vi "CRYProject Editor PART TS Write.vi"(7 "Channels":i32=2, 9 "Version":u16=1, 11 "pSaveName":path) -> (0 "Is Replace?":bool, 1 "SequenceFilepathOut":path, 2 "Sequence NameOut":string, 3 "status":bool, 4 "Flatten Doc Data":string, 5 "Flatten Curve Data":string)   [LabVIEW 2013]
uses:
  Control/CRYSequence Cluster.ctl
  CRYProject Editor Global.vi
  CRYSystem/Misc/SubVI/CRYMisc vis settings global.vi
  CRYMainGlobal.vi
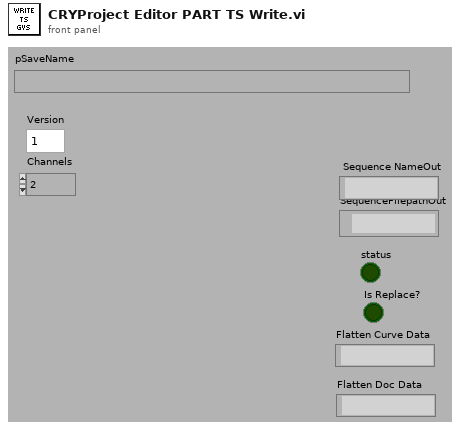
[diagram p1: front panel]
types:
  T1 = enum16{"New", "Open", "Close", "Close Data View Window Only", "Change", "Save", "Save for close"}
  T2 = typedef "CRYSequence Cluster.ctl" = cluster{"EditStepName":string, "Trimmed string array":string, "Flattened CurveData":string, "Document Data":string, "EditStepNo":u16, "Operator Start File":path, "Sequence Type":string, "Sequence Language":string, "Sequence Work State":string}
  T3 = enum16{"open", "replace", "create", "open or create", "replace or create", "replace or create with confirmation"}
  T4 = typedef "CRYTS.ctl" = cluster{"No.TS":u16, "TS File Path":path, "TS Name":string, "EditStepName":string, "Steps":T5[], "New State":bool, "Change State":bool, "Flattened CurveLib Data":string, "Document Data":string, "EditStepNo":u16, "Operator Start File":string, "Sequence Type":string, "Sequence Language":string}
  T5 = typedef "CRYStep.ctl" = cluster{"No.VI":i32, "Category":string, "StepName":string, "Seq setup flattened":string, "Comment":string, "Steps config.":bool[], "Jump config":i32[], "Start":dbl, "Increment":dbl, "Name":string, "Unit":string, "Y data":u16, "Y prefix":string, "Y dB ref":dbl, "Y unit":string, "Repeat State Array":cluster{"Start":dbl, "Increment":dbl, "Count":i32, "Num":i32}[]}
  T6 = enum32{"English", "Chinese", "Korean", "Japanese", "Russian", "Chinese traditional"}
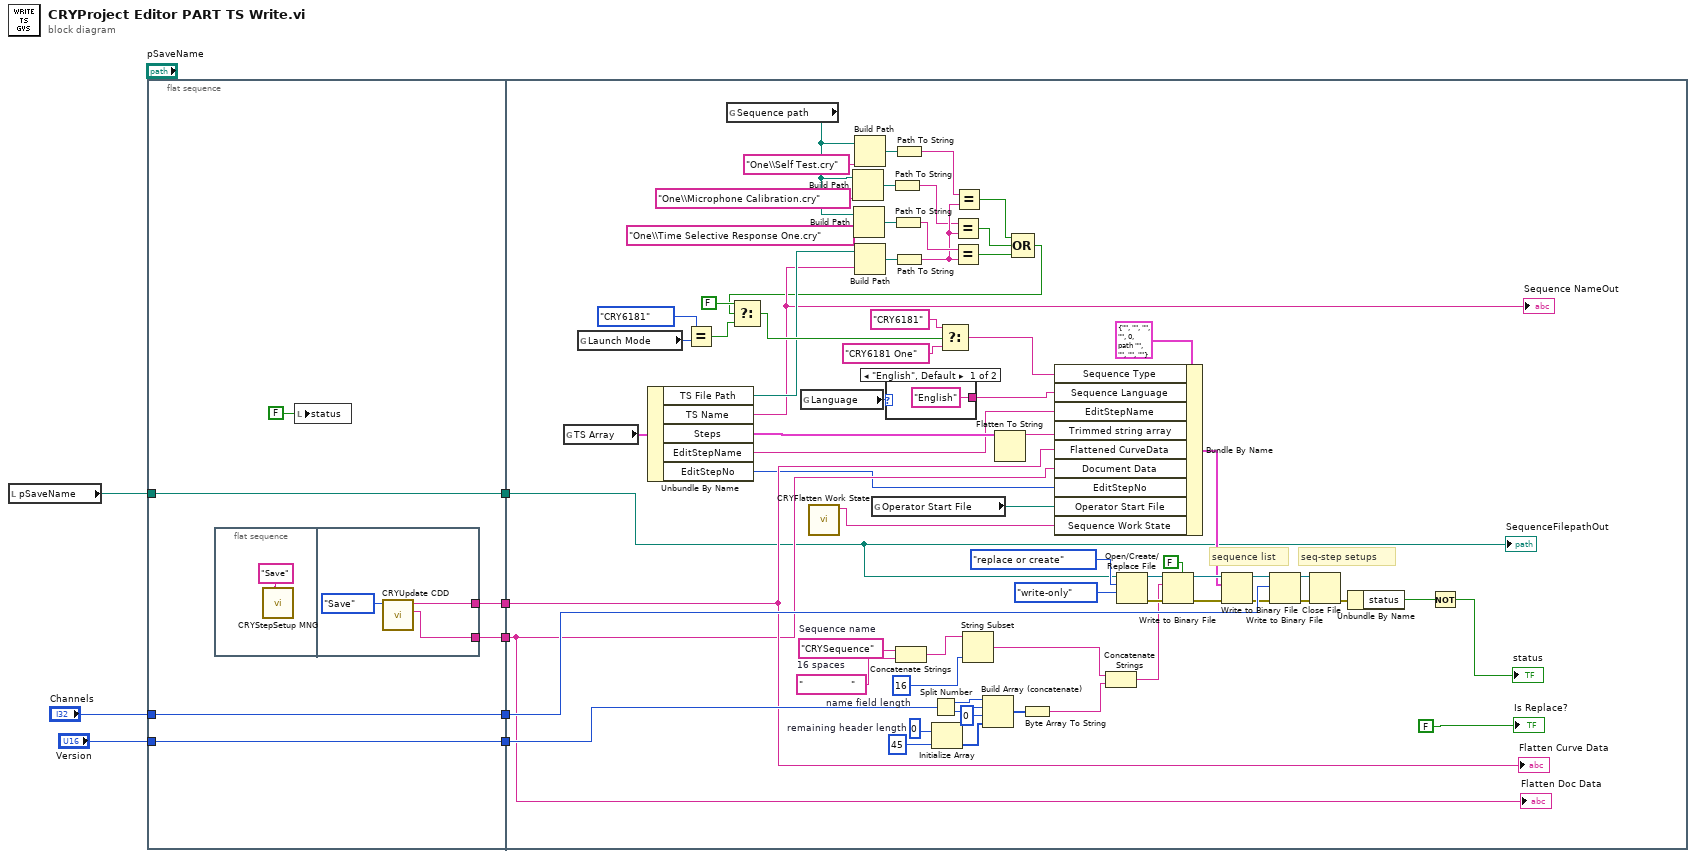
[diagram p0: block diagram]
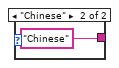
[diagram p2: hidden frame]
diagram:
  n1 = local read "pSaveName"() -> (w6:path)
  n2 = flat-sequence {
    tunnel: w6 -> [w12]
    tunnel: "Version" -> [w13]
    tunnel: "Channels" -> [w14]
    tunnel: [w14] -> w5
    tunnel: [w13] -> w4
    tunnel: [w10] -> w3
    tunnel: [w9] -> w2
    tunnel: [w12] -> w1
    tunnel: w5 -> [w88]
    tunnel: w4 -> [w87]
    tunnel: w3 -> [w84]
    tunnel: w2 -> [w83]
    tunnel: w1 -> [w51]
    frame #0 {
      n3 = flat-sequence {
        tunnel: [w16] -> w10
        tunnel: [w17] -> w9
        frame #0 {
          n4 = call "CRYStepSetup MNG.vi"("sAction"="Save" ("Option")) -> ()  [unwired: 9 in, 2 out]
        }
        frame #1 {
          n5 = call "CRYUpdate CDD.vi"("Signal"=T1."Save") -> ("Document Data Out"=w17:string, "Flatten Data Out"=w16:string)  [unwired: 2 in, 7 out]
        }
      }
      n6 = local write "status"(FALSE ("status")) -> ()
    }
    frame #1 {
      w63 = 16  # name field length
      w64 = "                "  # 16 spaces
      w65 = "CRYSequence"  # Sequence name
      w73 = 45  # remaining header length
      # "sequence list"
      # "seq-step setups"
      n7 = global read "CRYProject Editor Global.vi" "TS Array"() -> (w52:T4)
      n8 = global read "CRYMainGlobal.vi" "Launch Mode"() -> (w47:enum32{"CRY6181", "CRY6181 One"})
      n9 = Unbundle By Name(w52) -> ("TS File Path"=w37:path, "TS Name"=w36:string, "Steps"=w55:T5[], "EditStepName"=w53:string, "EditStepNo"=w50:u16)
      "Sequence NameOut" <- w36
      n10 = Equal?(x=enum32{"CRY6181", "CRY6181 One"}."CRY6181", y=w47) -> (x = y?=w44:bool)
      n11 = global read "CRYMainGlobal.vi" "Sequence path"() -> (w30:path)
      n12 = global read "CRYMainGlobal.vi" "Language"() -> (w22:T6)
      n13 = call "CRYFlatten Work State.vi"() -> ("work state # flattened"=w19:string)  [unwired: 11 in]
      n14 = Build Path(base path=w30, name or relative path="One\\Microphone Calibration.cry") -> (appended path=w34:path)
      n15 = Build Path(base path=w30, name or relative path="One\\Time Selective Response One.cry") -> (appended path=w40:path)
      n16 = Build Path(base path=w30, name or relative path="One\\Self Test.cry") -> (appended path=w31:path)
      n17 = Build Path(base path=w37, name or relative path=w36) -> (appended path=w39:path)
      n18 = global read "CRYMisc vis settings global.vi" "Operator Start File"() -> (w49:path)
      n19 = case shown="\"English\", Default" w22 {
        tunnel: ["English" ("TS Name") "Chinese" ("TS Name")] -> w20
        frame "English", Default {
        }
        frame "Chinese" {
        }
      }
      n20 = Path To String(path=w34) -> (string=w27:string)
      n21 = Path To String(path=w40) -> (string=w38:string)
      n22 = Path To String(path=w31) -> (string=w28:string)
      n23 = Path To String(path=w39) -> (string=w29:string)
      n24 = Concatenate Strings(w65, w64) -> (w62:string)
      n25 = Split Number(x=w87) -> (hi(x)=w58:u8, lo(x)=w57:u8)
      n26 = Initialize Array(u8 0, w73) -> (w72:u8[])
      n27 = Equal?(x=w27, y=w29) -> (x = y?=w26:bool)
      n28 = Equal?(x=w38, y=w29) -> (x = y?=w35:bool)
      n29 = Equal?(x=w28, y=w29) -> (x = y?=w25:bool)
      n30 = String Subset(string=w62, length (rest)=w63) -> (substring=w61:string)  [unwired: 1 out]
      n31 = Build Array (concatenate)(w58, w57, u8 0 ("element"), w72) -> (w71:u8[])
      n32 = Flatten To String(anything=w55) -> (data string=w54:string)  [unwired: 1 in, 4 out]
      n33 = Compound Arithmetic op=OR(w25, w26, w35) -> (w24:bool)
      n34 = Select(t=FALSE, s=w24, f=w44) -> (s? t:f=w42:bool)
      n35 = Select(t="CRY6181" ("Section"), s=w42, f="CRY6181 One" ("Section")) -> (s? t:f=w21:string)
      n36 = Byte Array To String(unsigned byte array=w71) -> (string=w60:string)
      n37 = Bundle By Name(cluster=T2 {"EditStepName"="", "Trimmed string array"="", "Flattened CurveData"="", "Document Data"="", "EditStepNo"=0, "Operator Start File"=path "", "Sequence Type"="", "Sequence Language"="", "Sequence Work State"=""} ("output cluster"), "Sequence Type"=w21, "Sequence Language"=w20, "EditStepName"=w53, "Trimmed string array"=w54, "Flattened CurveData"=w84, "Document Data"=w83, "EditStepNo"=w50, "Operator Start File"=w49, "Sequence Work State"=w19) -> (w66:T2)
      n38 = Concatenate Strings(w61, w60) -> (w59:string)
      n39 = Open/Create/Replace File(file path (use dialog)=w51, operation (0:open)=T3."replace or create", access (0:read/write)=enum16{"read/write", "read-only", "write-only"}."write-only") -> (refnum out=w78:refnum<file>, error out=w77:errorcluster)  [unwired: 1 in, 3 out]
      n40 = Write to Binary File(file (use dialog)=w78, data=w59, error in=w77, 5:FALSE ("prepend array or string size? (T)")) -> (error out=w76:errorcluster)  [unwired: 1 in, 3 out]
      n41 = Write to Binary File(file (use dialog)=w78, data=w66, error in=w76) -> (refnum out=w81:refnum<file>, error out=w82:errorcluster)  [unwired: 1 in, 3 out]
      n42 = Write to Binary File(file (use dialog)=w81, data=w88, error in=w82) -> (refnum out=w68:refnum<file>, error out=w67:errorcluster)  [unwired: 1 in, 3 out]
      n43 = Close File(refnum=w68, error in=w67) -> (error out=w70:errorcluster)  [unwired: 1 out]
      n44 = Unbundle By Name(w70) -> ("status"=w69:bool)
      n45 = Not(x=w69) -> (.not. x?=→"status":bool)
      "SequenceFilepathOut" <- w51
      "Is Replace?" <- FALSE ("Is Replace?")
      "Flatten Curve Data" <- w84
      "Flatten Doc Data" <- w83
    }
  }
